vi "Read CDBL.vi"(8 "error in (no error)":errorcluster, 10 "Tag":string, 11 "Var Bus in":refnum<class "Omni_Bus.lvclass">) -> (0 "error out":errorcluster, 2 "Numeric":cdb, 3 "Var Bus out":refnum<class "Omni_Bus.lvclass">)   [LabVIEW 2021, in "Omni_Bus.lvclass"]
uses:
  Omni_Bus.lvclass
  <vilib>/TSA/Abstract Data Classes/Abs_Types/Complex Double Float/Abs_Complex Double Float.lvclass
  Omni_Bus.lvclass/Omni_Bus.ctl
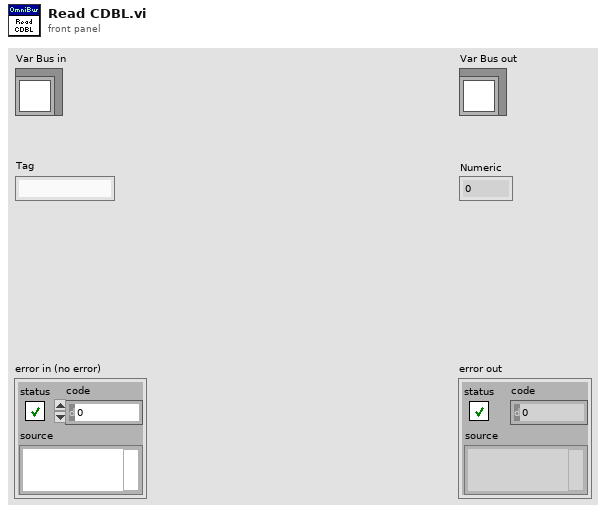
[diagram p1: front panel]
types:
  T1 = typedef "Abs_Complex Double Float.lvclass/Type.ctl" = cdb
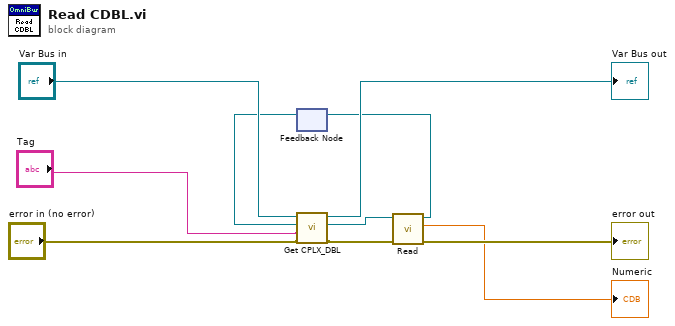
[diagram p0: block diagram]
diagram:
  n1 = feedback #1() -> (w1:refnum<class "Abs_Complex Double Float.lvclass">)  [unwired: 1 in]
  n2 = call-dynamic "Get CPLX_DBL.vi"("error in (no error)"="error in (no error)", "Tag"="Tag", "Value Type"=w1, "Var Bus in"="Var Bus in") -> ("error out"=w3:errorcluster, "Value Out"=w2:refnum<class "Abs_Complex Double Float.lvclass">, "Var Bus out"=→"Var Bus out":refnum<class "Omni_Bus.lvclass">)  [unwired: 5 in]
  n3 = call-dynamic "Read.vi"("error in (no error)"=w3, "Double Float.lvclass_340760 in"=w2) -> ("error out"=→"error out":errorcluster, "Value"=→"Numeric":T1, "Double Float.lvclass_340760 out"=w4:refnum<class "Abs_Complex Double Float.lvclass">)  [unwired: 7 in]
  n4 = feedback-in #1(w4) -> ()
